vi "RT-Main (BOTH).vi"() -> ()   [LabVIEW 2016]
uses:
  Update Screen.ctl
  Inventory FGV Command.ctl
  <vilib>/NI_Real-Time Target Support.lvlib
panel:
  in  "Stop Button 2":bool
  in  "Stop Button":bool
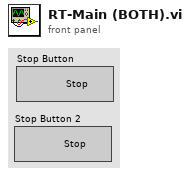
[diagram p1: front panel]
types:
  T1 = typedef "Update Screen.ctl" = cluster{"Time":string, "Item":string, "Name":string, "Action":string, "Lunch Names":string[]}
  T2 = typedef "Inventory FGV Command.ctl" = enum16{"Load Items", "Check Status", "Return Items", "Check Out Items", "Add New Item", "Get All Items", "Remove Item", "Search"}
  T3 = typedef "Array Device Info.ctl" = T4[]
  T4 = typedef "Device Info.ctl" = cluster{"Model Number":string, "Identifier":string, "Available?":bool, "Owner":string, "Owner Email":string, "Last Activity Date":string, "Loan Purpose":string, "Department":string, "Notes":string, "Serial Number":string}
  T5 = typedef "Array AE Data.ctl" = T6[]
  T6 = typedef "AE Data.ctl" = cluster{"Name":string, "Go?":bool, "Which batch?":enum16{"Anything", "First", "Second"}}
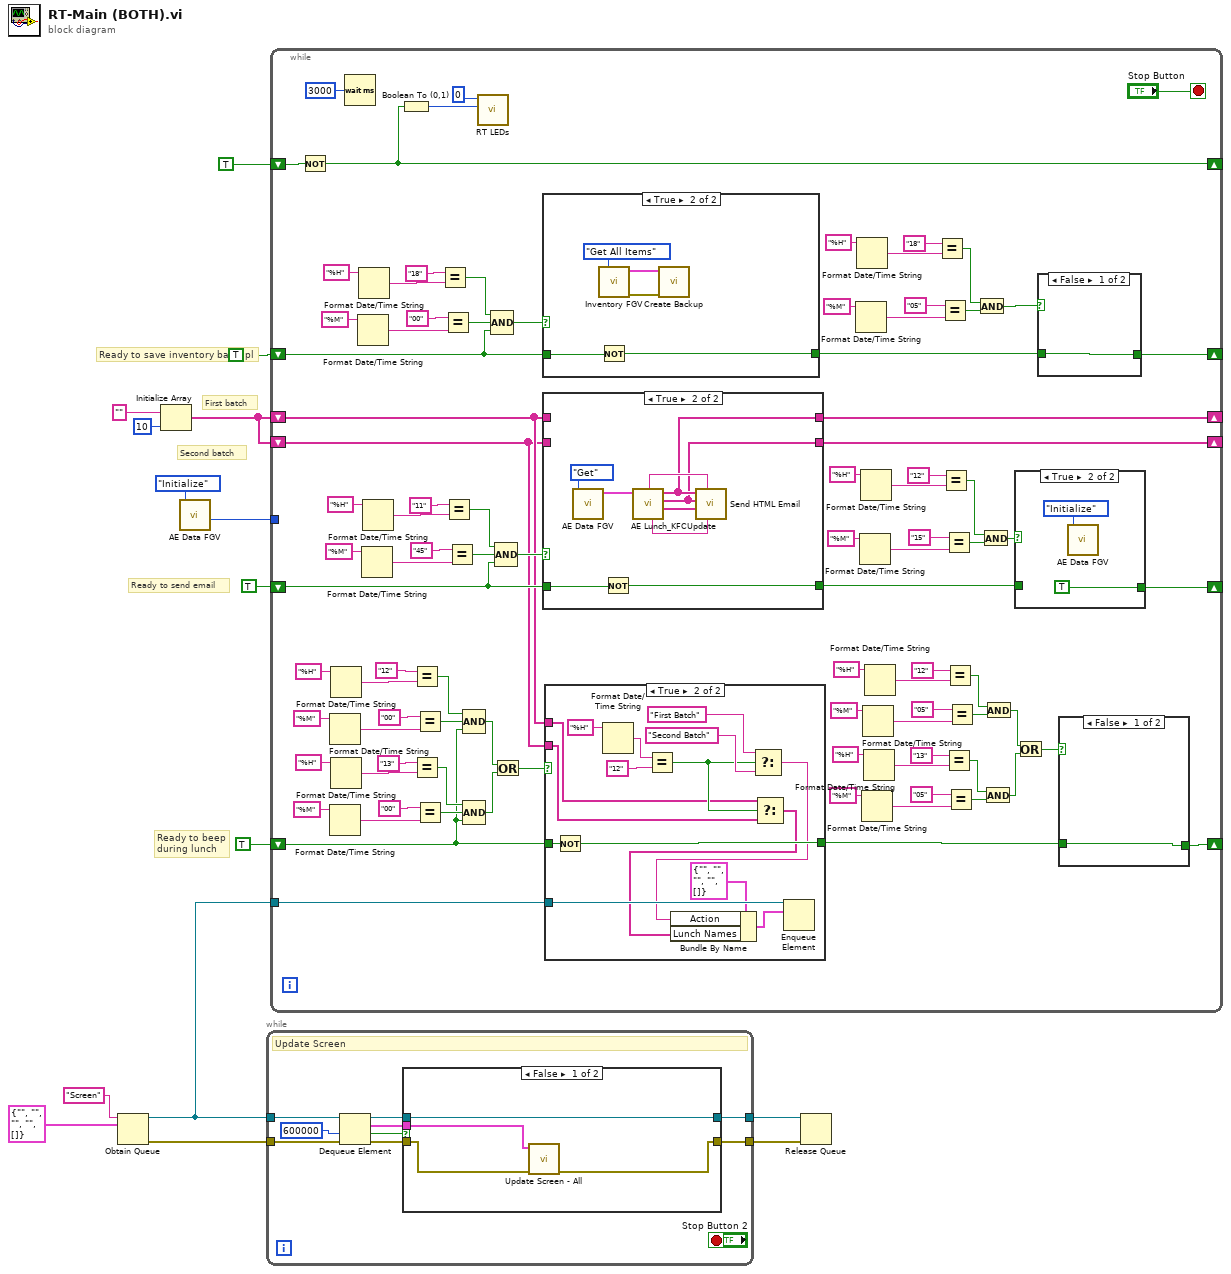
[diagram p0: block diagram]
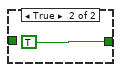
[diagram p4: hidden frame]
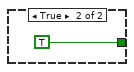
[diagram p6: hidden frame]
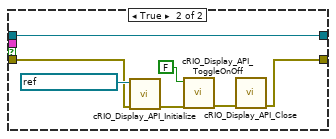
[diagram p8: hidden frame]
diagram:
  # "Second batch"
  # "First batch"
  # "Ready to beep\nduring lunch"
  # "Ready to send email"
  # "Ready to save inventory backupl"
  n1 = Obtain Queue(name (unnamed)="Screen", element data type=T1 {"Time"="", "Item"="", "Name"="", "Action"="", "Lunch Names"=[]}) -> (queue out=w1:refnum<queue>, error out=w12:errorcluster)  [unwired: 3 in, 1 out]
  n2 = Initialize Array("", 10 ("dimension size")) -> (w2:string[])
  n3 = call "AE Data FGV.vi"("Command"=enum16{"Initialize", "Update", "Get"}."Initialize") -> ("Index"=w7:i32)  [unwired: 9 in, 1 out]
  n4 = while {
    tunnel: w1 -> [w24]
    tunnel: w12 -> [w23]
    tunnel: [w17] -> w10
    tunnel: [w16] -> w9
    stop <- "Stop Button 2" stop-if-true
    # "Update Screen"
    n5 = Dequeue Element(queue=w24, timeout in ms (-1)=600000, error in (no error)=w23) -> (queue out=w18:refnum<queue>, element=w19:T1, timed out?=w21:bool, error out=w20:errorcluster)
    n6 = case shown="False" w21 {
      tunnel: w20 -> [w29 w32]
      tunnel: w19 -> [w26 _]
      tunnel: w18 -> [w27 w36]
      tunnel: [w28 w31] -> w17
      tunnel: [w27 w36] -> w16
      frame False {
        n7 = call "Update Screen - All.vi"("error in (no error)"=w29, "Update Screen"=w26) -> ("error out"=w28:errorcluster)  [unwired: 9 in]
      }
      frame True {
        n8 = call <vilib>:"cRIO_Display_API_Initialize.vi"("error in"=w32, "cRIODisplay Port"=refnum<visa-resource-name> "ASRL1::INSTR") -> ("error out"=w35:errorcluster)  [unwired: 9 in]
        n9 = call <vilib>:"cRIO_Display_API_ToggleOnOff.vi"("error in"=w35, "On/Off"=FALSE) -> ("error out"=w34:errorcluster)  [unwired: 9 in]
        n10 = call <vilib>:"cRIO_Display_API_Close.vi"("error in"=w34) -> ("error out"=w31:errorcluster)  [unwired: 10 in]
      }
    }
  }
  n11 = while {
    shift-right: [w128] -> _
    shift-left: TRUE -> [w129]
    shift-right: [w104] -> _
    shift-left: TRUE -> [w115]
    tunnel: w7 -> [_]
    shift-right: [w83] -> _
    shift-left: TRUE -> [w84]
    shift-right: [w65] -> _
    shift-left: TRUE -> [w56]
    shift-right: [w41] -> _
    shift-left: w2 -> [w39]
    shift-right: [w40] -> _
    shift-left: w2 -> [w38]
    tunnel: w1 -> [w37]
    stop <- "Stop Button" stop-if-true
    n12 = Not(x=w129) -> (.not. x?=w128:bool)
    n13 = Format Date/Time String(time format string (%c)="%M") -> (date/time string=w60:string)  [unwired: 2 in]
    n14 = Format Date/Time String(time format string (%c)="%M") -> (date/time string=w70:string)  [unwired: 2 in]
    n15 = Format Date/Time String(time format string (%c)="%H") -> (date/time string=w62:string)  [unwired: 2 in]
    n16 = Format Date/Time String(time format string (%c)="%H") -> (date/time string=w68:string)  [unwired: 2 in]
    n17 = Wait (ms)(milliseconds to wait=u32 3000) -> ()  [unwired: 1 out]
    n18 = Format Date/Time String(time format string (%c)="%M") -> (date/time string=w120:string)  [unwired: 2 in]
    n19 = Format Date/Time String(time format string (%c)="%H") -> (date/time string=w122:string)  [unwired: 2 in]
    n20 = Format Date/Time String(time format string (%c)="%M") -> (date/time string=w99:string)  [unwired: 2 in]
    n21 = Format Date/Time String(time format string (%c)="%H") -> (date/time string=w101:string)  [unwired: 2 in]
    n22 = Boolean To (0,1)(Boolean=w128) -> (0, 1=w127:i16)
    n23 = Equal?(x="12", y=w62) -> (x = y?=w58:bool)
    n24 = Equal?(x="13", y=w68) -> (x = y?=w72:bool)
    n25 = Equal?(x="00", y=w60) -> (x = y?=w57:bool)
    n26 = Equal?(x="00", y=w70) -> (x = y?=w73:bool)
    n27 = Equal?(x="18", y=w122) -> (x = y?=w118:bool)
    n28 = Equal?(x="00", y=w120) -> (x = y?=w117:bool)
    n29 = Equal?(x="11", y=w101) -> (x = y?=w97:bool)
    n30 = Equal?(x="45", y=w99) -> (x = y?=w96:bool)
    n31 = Compound Arithmetic op=AND(w58, w57, w56) -> (w55:bool)
    n32 = Compound Arithmetic op=AND(w72, w73, w56) -> (w54:bool)
    n33 = call <vilib>:"RT LEDs.vi"("State"=w127, "LED Num"=0) -> ()  [unwired: 4 in, 2 out]
    n34 = Compound Arithmetic op=AND(w118, w117, w115) -> (w116:bool)
    n35 = Or(x=w55, y=w54) -> (x .or. y?=w53:bool)
    n36 = Compound Arithmetic op=AND(w97, w96, w84) -> (w95:bool)
    n37 = case shown="True" w116 {
      tunnel: w115 -> [w143 w148]
      tunnel: [w143 w147] -> w105
      frame False {
      }
      frame True {
        n38 = call "Inventory FGV.vi"("Command"=Inventory_FGV_Command."Get All Items") -> ("error out"=w144:errorcluster, "array of devices"=w145:T3)  [unwired: 7 in, 1 out]
        n39 = Not(x=w148) -> (.not. x?=w147:bool)
        n40 = call "Create Backup.vi"("error in"=w144, "array of devices"=w145) -> ()  [unwired: 9 in, 1 out]
      }
    }
    n41 = case shown="True" w95 {
      tunnel: w84 -> [w133 w142]
      tunnel: [w133 w141] -> w85
      tunnel: [w132 w135] -> w41
      tunnel: w39 -> [w132 _]
      tunnel: [w131 w134] -> w40
      tunnel: w38 -> [w131 _]
      frame False {
      }
      frame True {
        n42 = call "AE Data FGV.vi"("Command"=enum16{"Initialize", "Update", "Get"}."Get") -> ("Array of AEs"=w139:T5)  [unwired: 9 in, 1 out]
        n43 = Not(x=w142) -> (.not. x?=w141:bool)
        n44 = call "AE Lunch_KFCUpdate.vi"("Array of AEs"=w139) -> ("Not Going"=w138:string[], "Second Batch"=w134:string[], "First Batch"=w135:string[], "Second Batch Food"=w136:string, "First Batch Food"=w137:string)  [unwired: 6 in]
        n45 = call "Send HTML Email.vi"("Second Batch Food"=w136, "First Batch Food"=w137, "Not Going"=w138, "Second Batch"=w134, "First Batch"=w135) -> ()  [unwired: 5 in, 2 out]
      }
    }
    n46 = case shown="True" w53 {
      tunnel: w56 -> [w151 w166]
      tunnel: [w151 w165] -> w82
      tunnel: w39 -> [_ w156]
      tunnel: w38 -> [_ w155]
      tunnel: w37 -> [_ w164]
      frame False {
      }
      frame True {
        n47 = Not(x=w166) -> (.not. x?=w165:bool)
        n48 = Format Date/Time String(time format string (%c)="%H") -> (date/time string=w162:string)  [unwired: 2 in]
        n49 = Equal?(x=w162, y="12" ("x")) -> (x = y?=w157:bool)
        n50 = Select(t="First Batch", s=w157, f="Second Batch") -> (s? t:f=w154:string)
        n51 = Select(t=w156, s=w157, f=w155) -> (s? t:f=w153:string[])
        n52 = Bundle By Name(cluster=T1 {"Time"="", "Item"="", "Name"="", "Action"="", "Lunch Names"=[]}, "Action"=w154, "Lunch Names"=w153) -> (w152:T1)
        n53 = Enqueue Element(queue=w164, element=w152) -> ()  [unwired: 2 in, 3 out]
      }
    }
    n54 = Format Date/Time String(time format string (%c)="%M") -> (date/time string=w113:string)  [unwired: 2 in]
    n55 = Format Date/Time String(time format string (%c)="%H") -> (date/time string=w111:string)  [unwired: 2 in]
    n56 = Format Date/Time String(time format string (%c)="%M") -> (date/time string=w93:string)  [unwired: 2 in]
    n57 = Format Date/Time String(time format string (%c)="%H") -> (date/time string=w91:string)  [unwired: 2 in]
    n58 = Format Date/Time String(time format string (%c)="%M") -> (date/time string=w75:string)  [unwired: 2 in]
    n59 = Format Date/Time String(time format string (%c)="%M") -> (date/time string=w51:string)  [unwired: 2 in]
    n60 = Format Date/Time String(time format string (%c)="%H") -> (date/time string=w77:string)  [unwired: 2 in]
    n61 = Format Date/Time String(time format string (%c)="%H") -> (date/time string=w49:string)  [unwired: 2 in]
    n62 = Equal?(x="18", y=w111) -> (x = y?=w108:bool)
    n63 = Equal?(x="05", y=w113) -> (x = y?=w107:bool)
    n64 = Equal?(x="12", y=w91) -> (x = y?=w88:bool)
    n65 = Equal?(x="15", y=w93) -> (x = y?=w87:bool)
    n66 = Equal?(x="13", y=w77) -> (x = y?=w80:bool)
    n67 = Equal?(x="12", y=w49) -> (x = y?=w46:bool)
    n68 = Equal?(x="05", y=w75) -> (x = y?=w81:bool)
    n69 = Equal?(x="05", y=w51) -> (x = y?=w45:bool)
    n70 = And(x=w108, y=w107) -> (x .and. y?=w106:bool)
    n71 = And(x=w88, y=w87) -> (x .and. y?=w86:bool)
    n72 = And(x=w80, y=w81) -> (x .and. y?=w43:bool)
    n73 = And(x=w46, y=w45) -> (x .and. y?=w44:bool)
    n74 = case shown="True" w86 {
      tunnel: w85 -> [w169 _]
      tunnel: [w169 TRUE] -> w83
      frame False {
      }
      frame True {
        n75 = call "AE Data FGV.vi"("Command"=enum16{"Initialize", "Update", "Get"}."Initialize") -> ()  [unwired: 9 in, 2 out]
      }
    }
    n76 = Or(x=w44, y=w43) -> (x .or. y?=w42:bool)
    n77 = case shown="False" w106 {
      tunnel: w105 -> [w149 _]
      tunnel: [w149 TRUE] -> w104
      frame False {
      }
      frame True {
      }
    }
    n78 = case shown="False" w42 {
      tunnel: w82 -> [w167 _]
      tunnel: [w167 TRUE] -> w65
      frame False {
      }
      frame True {
      }
    }
  }
  n79 = Release Queue(queue=w9, error in (no error)=w10) -> ()  [unwired: 1 in, 3 out]
